vi "JSON_TTLConnect.vi"(0 "port":u16=5557, 1 "channel":u16, 2 "identifier":string, 3 "error in":errorcluster, 4 "highest channel":i32=8) -> (5 "context out":refnum<class "zmq_context.lvclass">, 6 "socket out":refnum<class "zmq_socket.lvclass">, 7 "error out":errorcluster)   [LabVIEW 2017]
doc: "Opens a ZeroMQ socket and subscribes to OpenEphys TTL events."
uses:
  <vilib>/addons/zeromq/zmq_socket.lvclass
  <vilib>/addons/zeromq/zmq_context.lvclass
  <vilib>/addons/zeromq/socket_type.ctl
  <vilib>/addons/zeromq/socket_options.ctl
  <vilib>/addons/zeromq/zeromq.lvlib
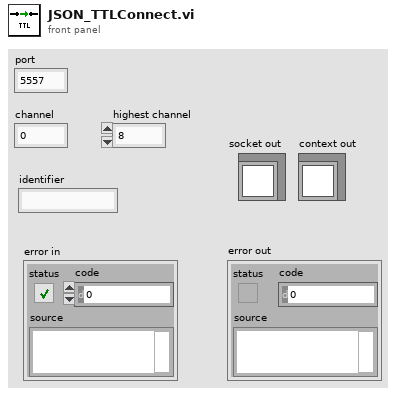
[diagram p1: front panel]
types:
  T1 = typedef "zeromq.lvlib/socket_type.ctl" = enum8{"ZMQ_PAIR", "ZMQ_PUB", "ZMQ_SUB", "ZMQ_REQ", "ZMQ_REP", "ZMQ_DEALER", "ZMQ_ROUTER", "ZMQ_PULL", "ZMQ_PUSH", "ZMQ_XPUB", "ZMQ_XSUB"}
  T2 = typedef "zeromq.lvlib/socket_options.ctl" = enum8{"NONE", "ZMQ_HWM", "<2>", "ZMQ_SWAP", "ZMQ_AFFINITY", "ZMQ_IDENTITY", "ZMQ_SUBSCRIBE", "ZMQ_UNSUBSCRIBE", "ZMQ_RATE", "ZMQ_RECOVERY_IVL", "ZMQ_MCAST_LOOP", "ZMQ_SNDBUF", "ZMQ_RCVBUF", "ZMQ_RCVMORE", "ZMQ_FD", "ZMQ_EVENTS", "ZMQ_TYPE", "ZMQ_LINGER", "ZMQ_RECONNECT_IVL", "ZMQ_BACKLOG", "ZMQ_RECOVERY_IVL_MSEC", "ZMQ_RECONNECT_IVL_MAX", "ZMQ_MAXMSGSIZE", "ZMQ_SNDHWM", "ZMQ_RCVHWM", "ZMQ_MULTICAST_HOPS", "<26>", "ZMQ_RCVTIMEO", "ZMQ_SNDTIMEO", "<29>", "<30>", "ZMQ_IPV4ONLY", "ZMQ_LAST_ENDPOINT", "ZMQ_ROUTER_MANDATORY", "ZMQ_TCP_KEEPALIVE", "ZMQ_TCP_KEEPALIVE_CNT", "ZMQ_TCP_KEEPALIVE_IDLE", "ZMQ_TCP_KEEPALIVE_INTVL", "ZMQ_TCP_ACCEPT_FILTER", "ZMQ_DELAY_ATTACH_ON_CONNECT", "ZMQ_XPUB_VERBOSE"}
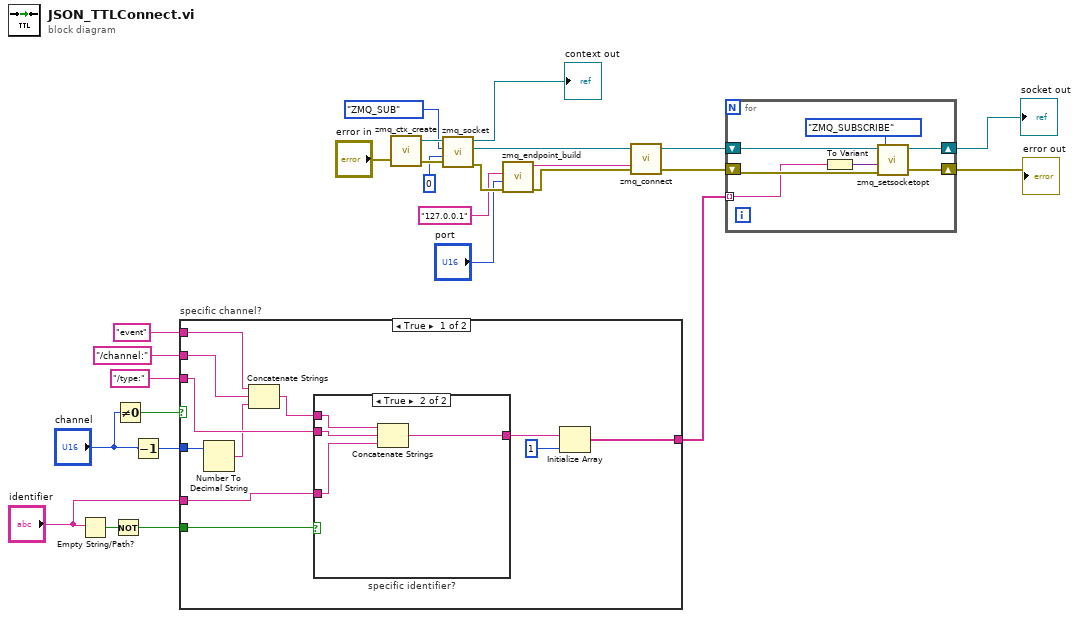
[diagram p0: block diagram]
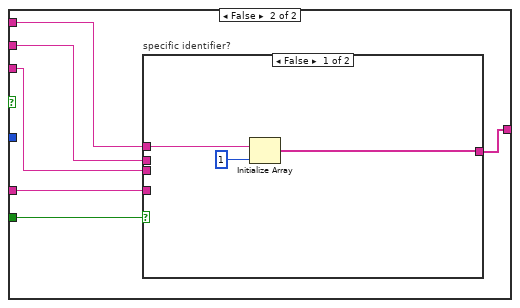
[diagram p3: hidden frame]
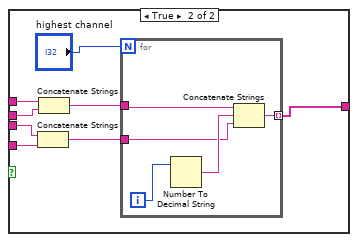
[diagram p4: hidden frame]
diagram:
  n1 = Empty String/Path?(string/path="identifier") -> (empty?=w9:bool)
  n2 = Not(x=w9) -> (.not. x?=w8:bool)
  n3 = Not Equal To 0?(x="channel") -> (x != 0?=w10:bool)
  n4 = Decrement(x="channel") -> (x-1=w3:u16)
  n5 = case "specific channel?" shown="True" w10 {
    tunnel: w3 -> [w36 _]
    tunnel: w8 -> [w37 w48]
    tunnel: "event" -> [w34 w47]
    tunnel: "/channel:" -> [w33 w45]
    tunnel: "/type:" -> [w35 w44]
    tunnel: "identifier" -> [w30 w43]
    tunnel: [w27 w46] -> w1
    frame True {
      n6 = Number To Decimal String(number=w36) -> (decimal integer string=w32:string)  [unwired: 1 in]
      n7 = Concatenate Strings(w34, w33, w32) -> (w31:string)
      n8 = case "specific identifier?" shown="True" w37 {
        tunnel: w35 -> [_ w41]
        tunnel: w31 -> [w38 w42]
        tunnel: w30 -> [_ w40]
        tunnel: [w38 w39] -> w28
        frame False {
        }
        frame True {
          n9 = Concatenate Strings(w42, w41, w40) -> (w39:string)
        }
      }
      n10 = Initialize Array(w28, 1 ("dimension size")) -> (w27:string[])
    }
    frame False {
      n11 = case "specific identifier?" shown="False" w48 {
        tunnel: w47 -> [w50 w58]
        tunnel: [w49 w52] -> w46
        tunnel: w45 -> [_ w57]
        tunnel: w44 -> [_ w54]
        tunnel: w43 -> [_ w55]
        frame False {
          n12 = Initialize Array(w50, 1 ("dimension size")) -> (w49:string[])
        }
        frame True {
          n13 = Concatenate Strings(w54, w55) -> (w53:string)
          n14 = Concatenate Strings(w58, w57) -> (w56:string)
          n15 = for {
            N: "highest channel" -> [_]
            tunnel: w56 -> [w64]
            tunnel: w53 -> [w62]
            tunnel: [w61] -> w52 mode=indexing
            i -> [w60]
            n16 = Number To Decimal String(number=w60) -> (decimal integer string=w63:string)  [unwired: 1 in]
            n17 = Concatenate Strings(w64, w63, w62) -> (w61:string)
          }
        }
      }
    }
  }
  n18 = call <vilib>:"zmq_ctx_create.vi"("error in"="error in") -> ("error out"=w26:errorcluster, "context out"=w25:refnum<class "zmq_context.lvclass">)  [unwired: 3 in]
  n19 = call <vilib>:"zmq_socket.vi"("error in"=w26, "linger (ms)"=0, "socket type"=socket_type."ZMQ_SUB", "context in"=w25) -> ("error out"=w19:errorcluster, "socket out"=w20:refnum<class "zmq_socket.lvclass">, "context out"=→"context out":refnum<class "zmq_context.lvclass">)  [unwired: 1 in]
  n20 = call <vilib>:"zmq_endpoint_build.vi"("error in"=w19, "port"="port", "address"="127.0.0.1" ("initial string")) -> ("error out"=w15:errorcluster, "endpoint"=w16:string)  [unwired: 2 in, 1 out]
  n21 = call <vilib>:"zmq_connect.vi"("error in"=w15, "endpoint"=w16, "socket in"=w20) -> ("error out"=w11:errorcluster, "socket out"=w22:refnum<class "zmq_socket.lvclass">)  [unwired: 1 in]
  n22 = for {
    shift-right: [w67] -> w13
    shift-left: w22 -> [w70]
    shift-right: [w68] -> w14
    shift-left: w11 -> [w66]
    tunnel: w1 -> [w65] mode=indexing
    n23 = To Variant(anything=w65) -> (Variant=w69:variant)
    n24 = call <vilib>:"zmq_setsocketopt.vi"("error in"=w66, "value"=w69, "option"=socket_options."ZMQ_SUBSCRIBE", "socket in"=w70) -> ("error out"=w68:errorcluster, "socket out"=w67:refnum<class "zmq_socket.lvclass">)  [unwired: 2 in]
  }
  "error out" <- w14
  "socket out" <- w13
